vi "zad1.vi"() -> ()   [LabVIEW 2017]
panel:
  out "Wynik":dbl
  in  "b":dbl
  in  "a":dbl
  # "a"
  # "b"
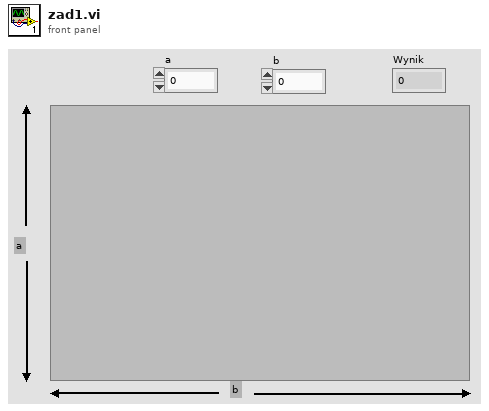
[diagram p1: front panel]
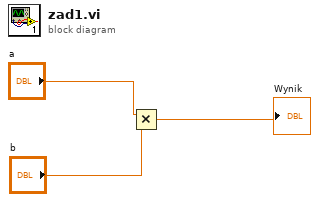
[diagram p0: block diagram]
diagram:
  n1 = Multiply(x="a", y="b") -> (x*y=→"Wynik":dbl)
